vi "iPSset.vi"(7 "Field Rate, T/min":dbl, 8 "error in (no error)":errorcluster, 9 "Target Field, T":dbl, 10 "iPSSetCtrl":T1, 11 "VISA resource name":refnum<visa-resource-name>) -> (0 "error out":errorcluster, 1 "read buffer":string, 2 "number":dbl, 3 "VISA resource name out":refnum<visa-resource-name>)   [LabVIEW 2021]
uses:
  controls/iPSsetCtrl.ctl
  <vilib>/regexp/Match Regular Expression.xnode
panel:
  out "call chain":string[](array[string])
  out "concatenated string 2":string
  out "concatenated string":string
  out "after match":string
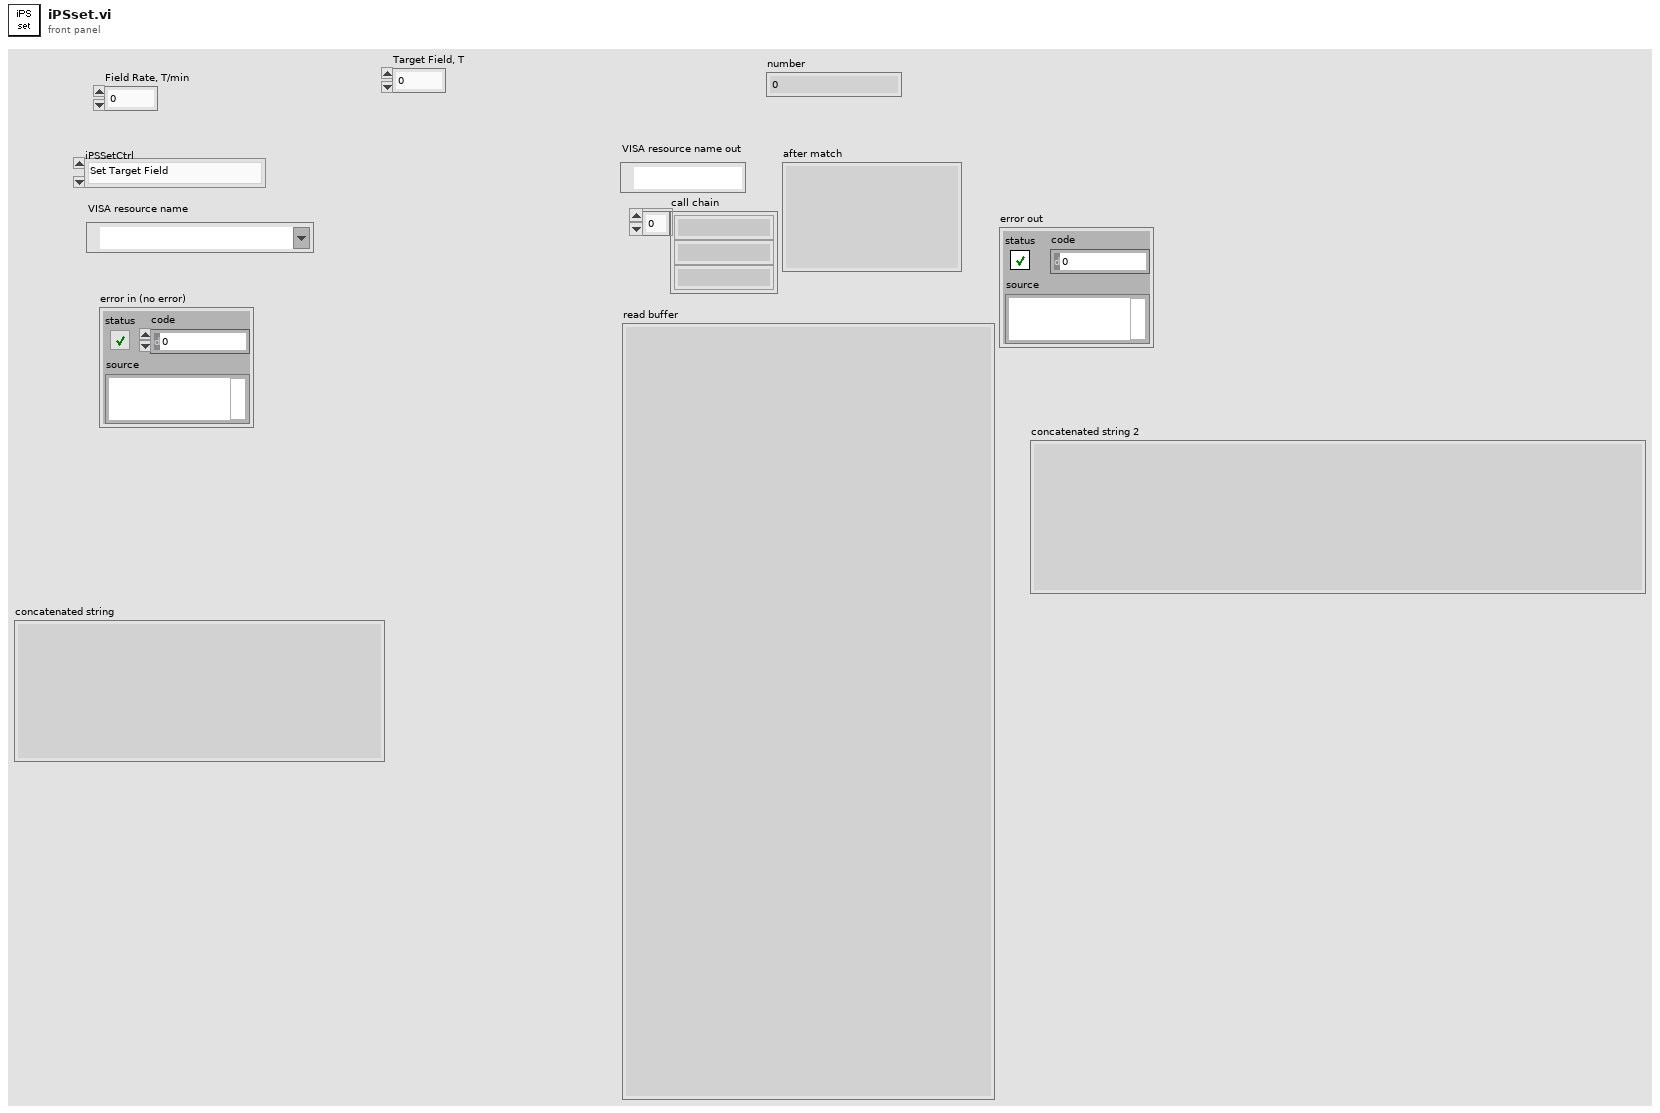
[diagram p1: front panel]
types:
  T1 = typedef "iPSsetCtrl.ctl" = enum16{"Set Target Field", "Set Target Field Rate", "Switch Heater ON", "Switch Heater OFF", "Go to Field", "Go to Zero", "Hold"}
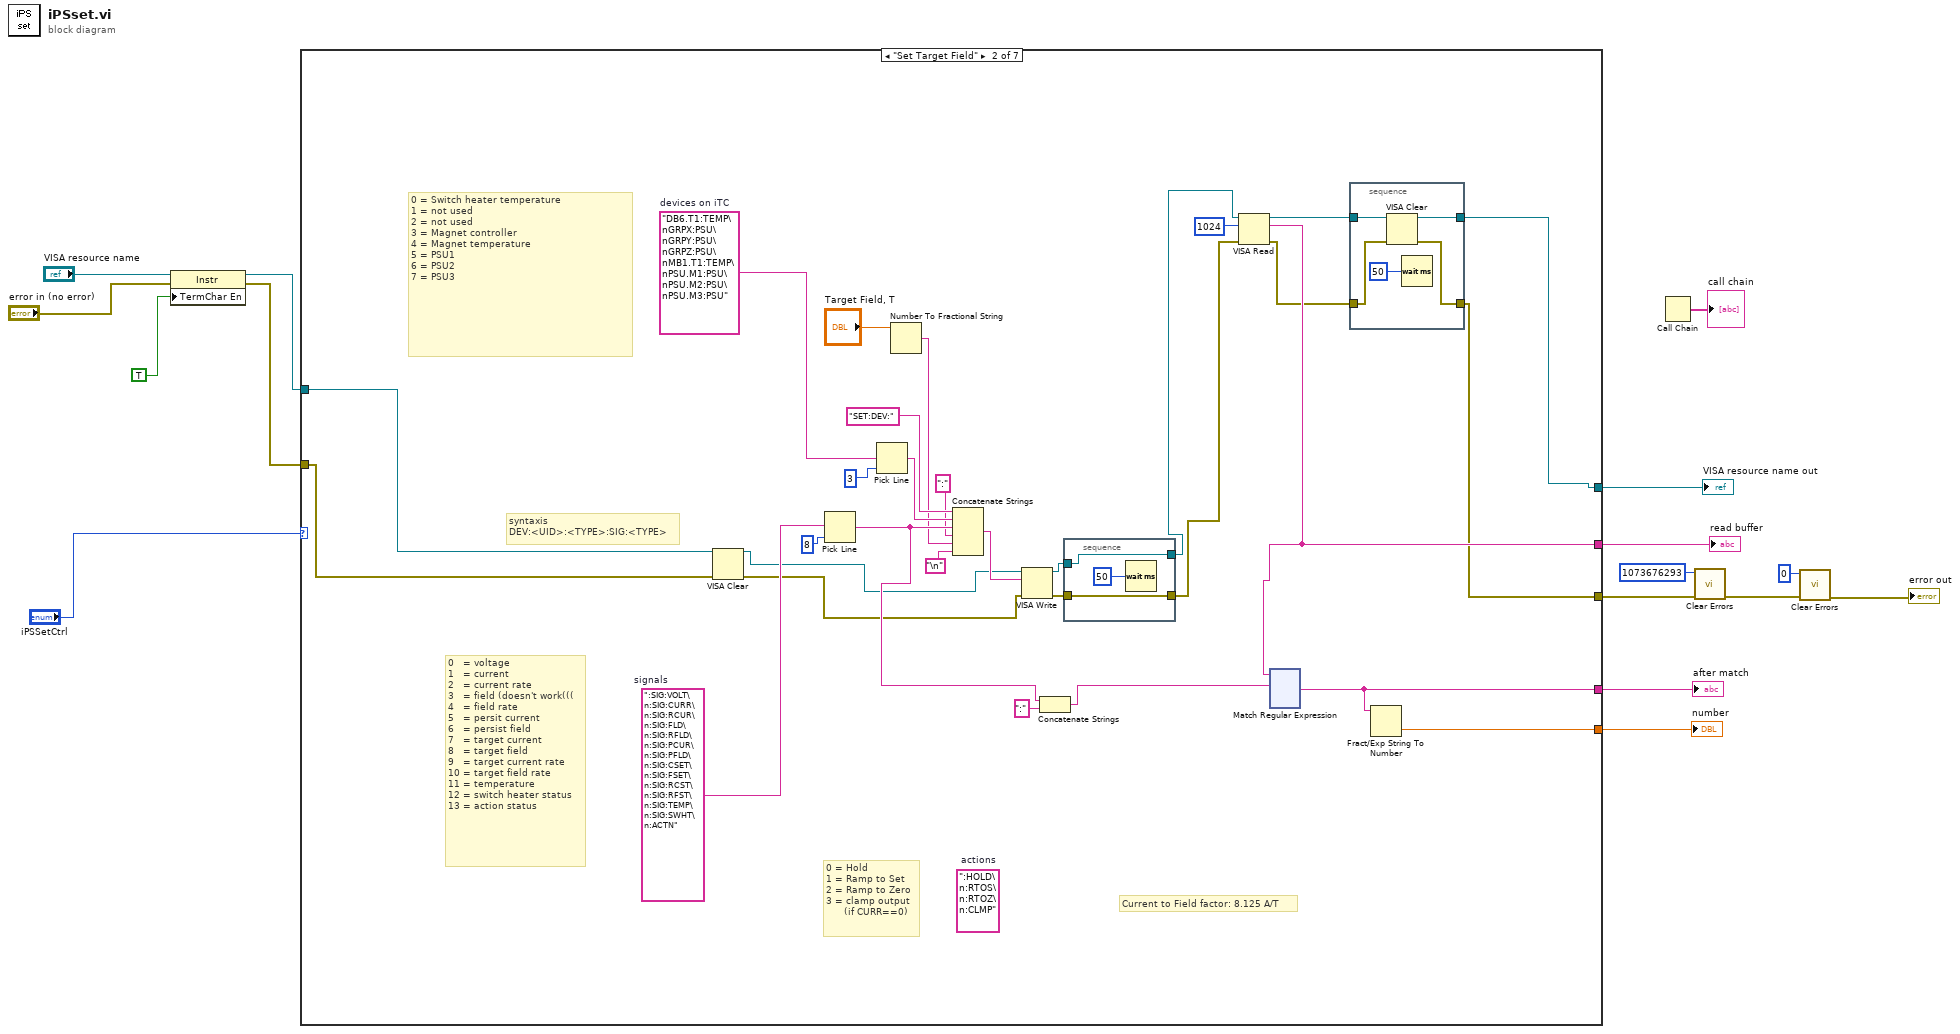
[diagram p0: block diagram]
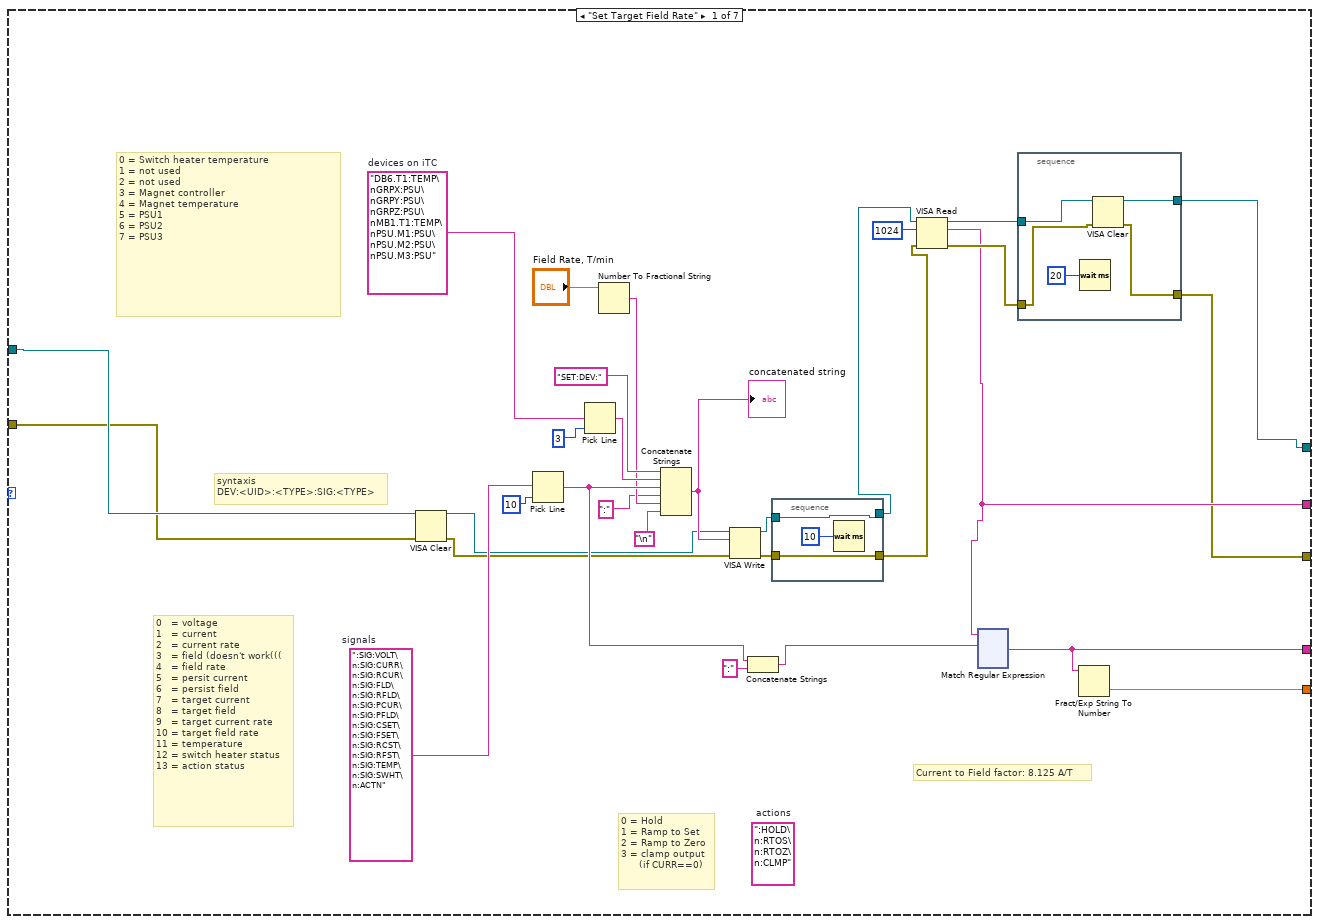
[diagram p2: hidden frame]
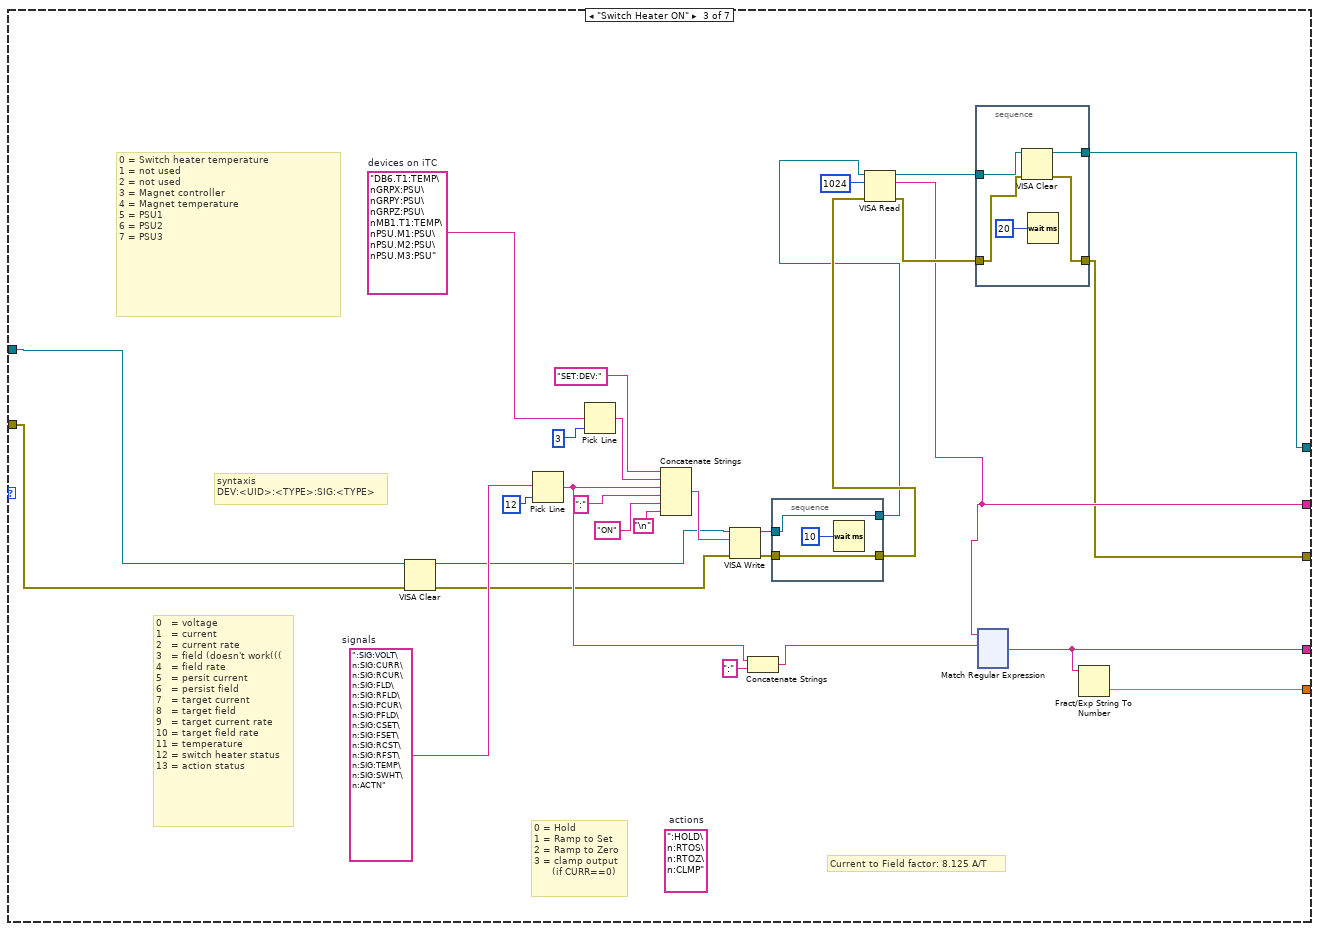
[diagram p3: hidden frame]
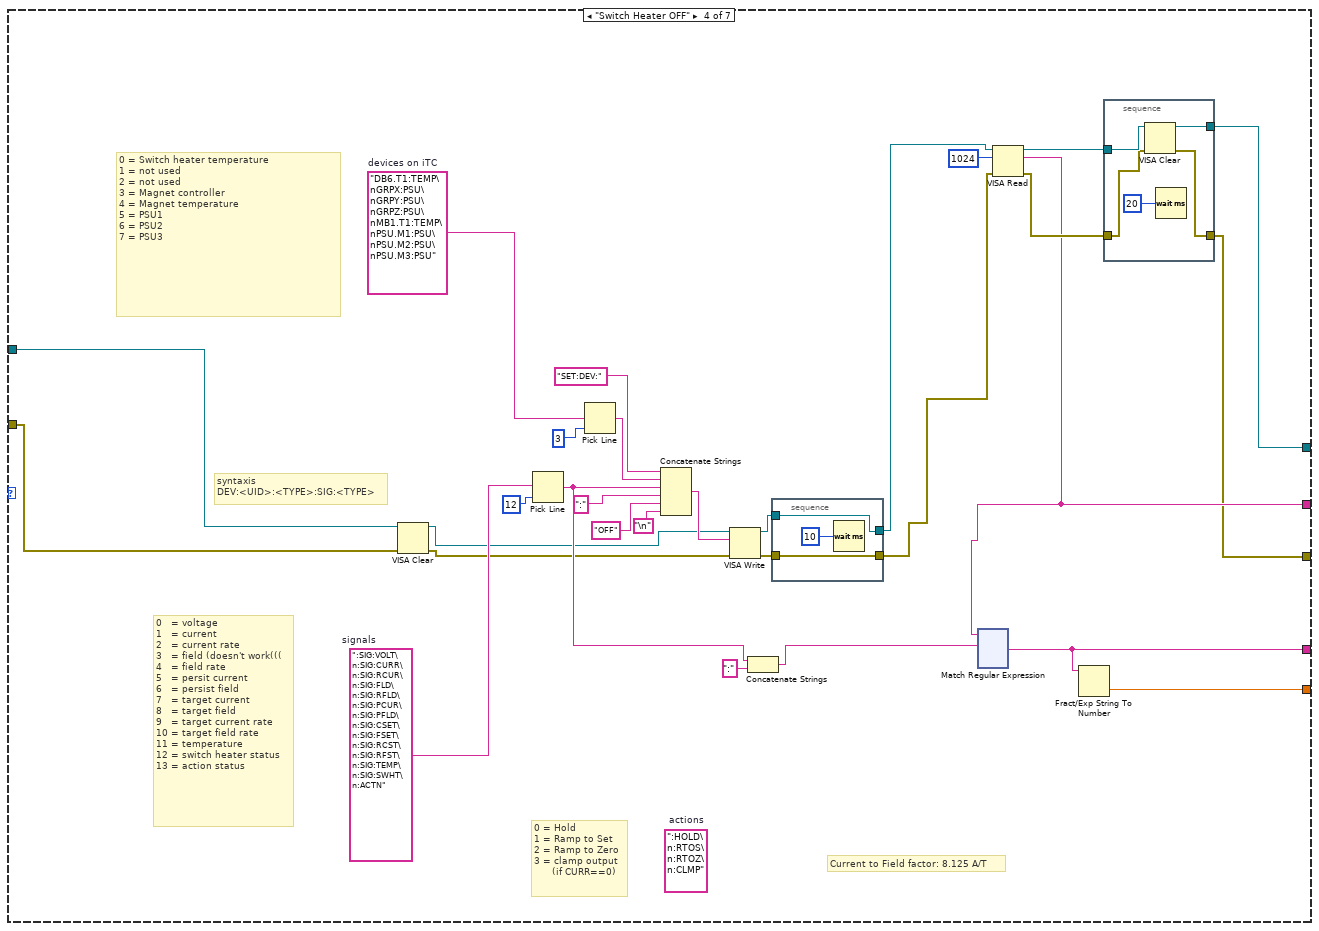
[diagram p4: hidden frame]
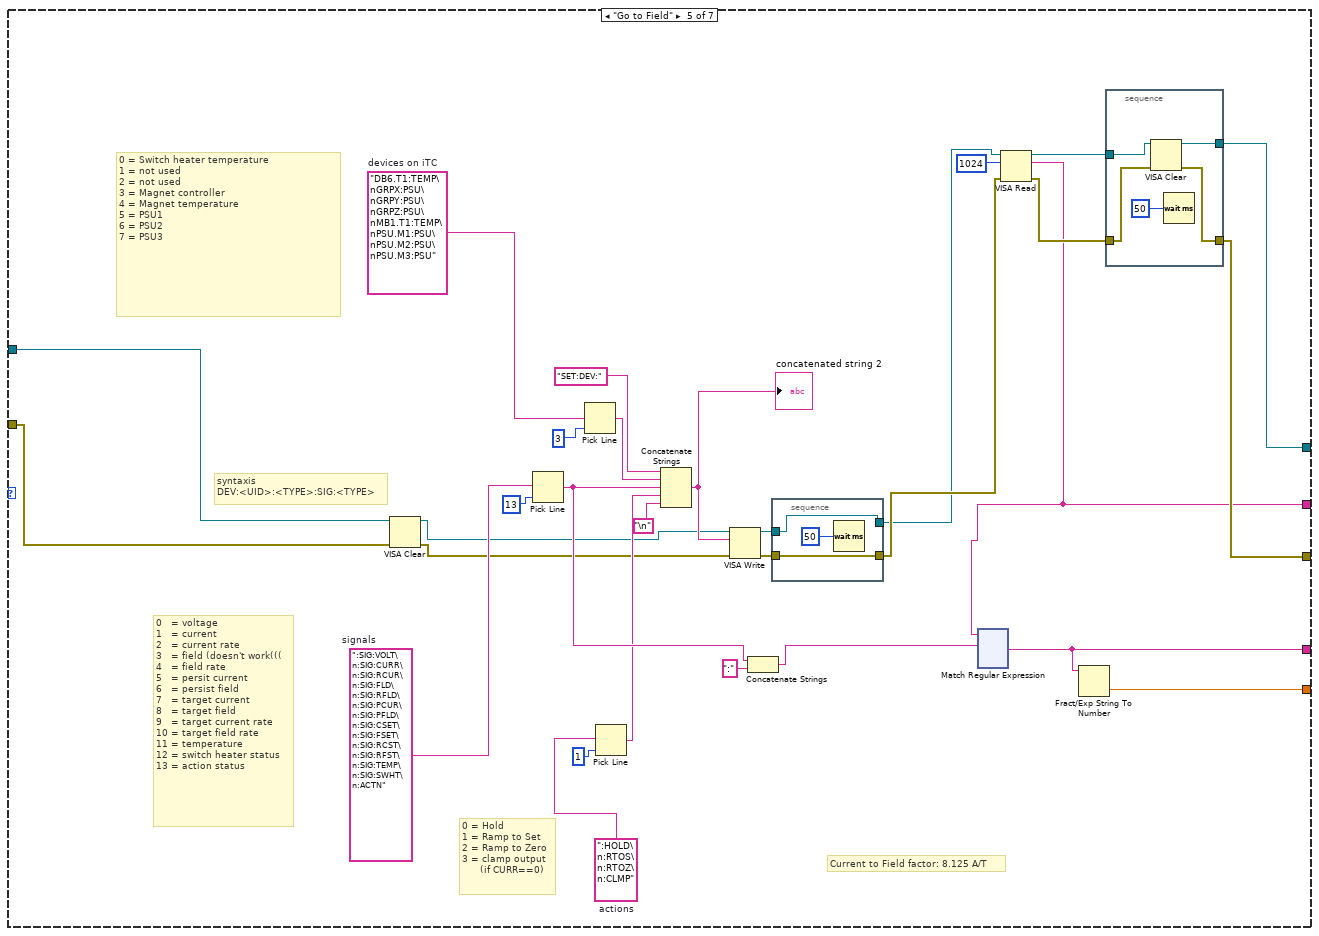
[diagram p5: hidden frame]
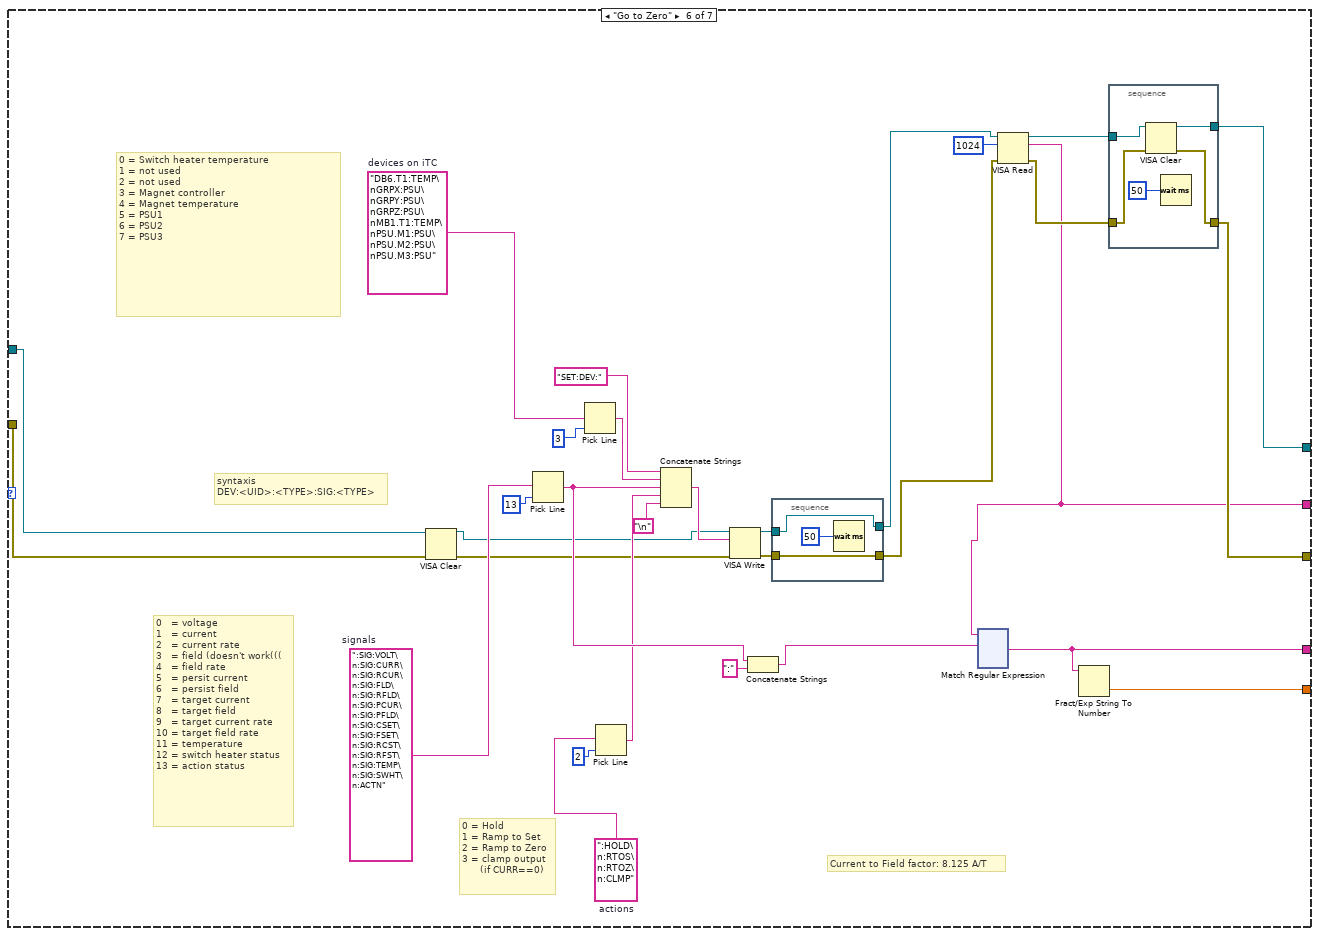
[diagram p6: hidden frame]
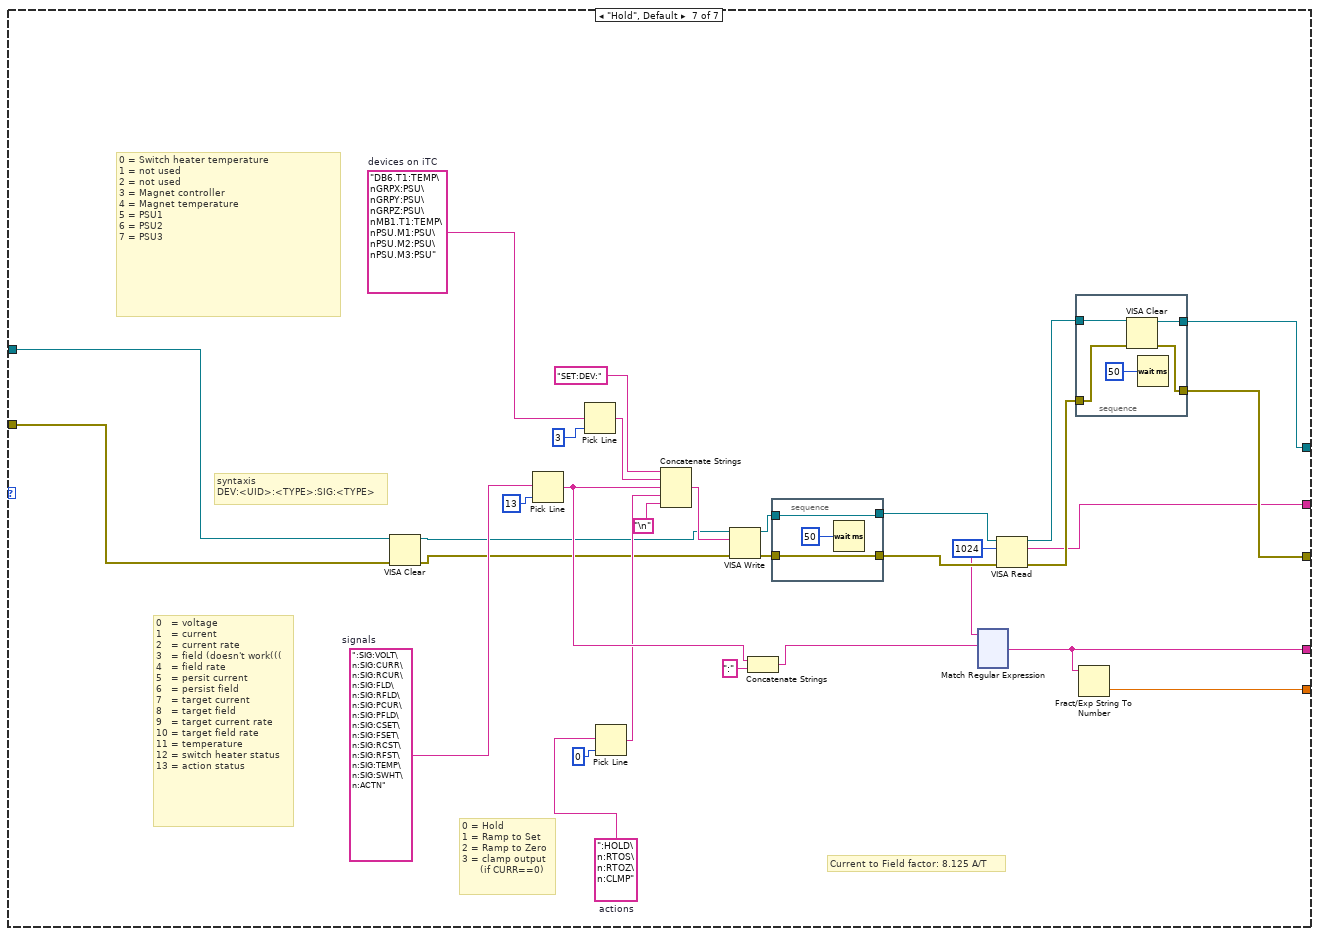
[diagram p7: hidden frame]
diagram:
  n1 = property class="Instr"(reference="VISA resource name", error in="error in (no error)", "TermChar En"=TRUE ("Message Based Settings:Termination Character Enable")) -> (reference out=w10:refnum<visa-resource-name>, error out=w9:errorcluster)
  n2 = case shown="\"Set Target Field\"" "iPSSetCtrl" {
    tunnel: [w25 w180 w335 w489 w645 w800 w954] -> w6
    tunnel: [w19 w174 w329 w483 w637 w793 w947] -> w16
    tunnel: [w26 w182 w336 w490 w644 w798 w953] -> w15
    tunnel: [w36 w191 w345 w499 w654 w809 w964] -> w14
    tunnel: [w35 w190 w344 w498 w653 w808 w963] -> w13
    tunnel: w9 -> [w23 w178 w333 w488 w642 w797 w952]
    tunnel: w10 -> [w24 w179 w334 w485 w640 w794 w949]
    frame "Set Target Field Rate" {
      (unwired) ":HOLD\n:RTOS\n:RTOZ\n:CLMP"  # actions
      w41 = ":SIG:VOLT\n:SIG:CURR\n:SIG:RCUR\n:SIG:FLD\n:SIG:RFLD\n:SIG:PCUR\n:SIG:PFLD\n:SIG:CSET\n:SIG:FSET\n:SIG:RCST\n:SIG:RFST\n:SIG:TEMP\n:SIG:SWHT\n:ACTN"  # signals
      w46 = "DB6.T1:TEMP\nGRPX:PSU\nGRPY:PSU\nGRPZ:PSU\nMB1.T1:TEMP\nPSU.M1:PSU\nPSU.M2:PSU\nPSU.M3:PSU"  # devices on iTC
      # "0 = Hold\n1 = Ramp to Set\n2 = Ramp to Zero\n3 = clamp output\n      (if CURR==0)"
      # "Current to Field factor: 8.125 A/T"
      # "0 = Switch heater temperature\n1 = not used\n2 = not used\n3 = Magnet controller \n4 = Magnet temperature\n5 = PSU1 \n6 = PSU2\n7 = PSU3"
      # "0   = voltage\n1   = current\n2   = current rate\n3   = field (doesn't work(((\n4   = field rate\n5   = persit current\n6   = persist field\n7   = target current\n8   = target field\n9   = target current rate\n10 = target field rate \n11 = temperature\n12 = switch heater status\n13 = action status"
      # "syntaxis\nDEV:<UID>:<TYPE>:SIG:<TYPE>"
      n3 = VISA Clear(VISA resource name=w24, error in (no error)=w23) -> (VISA resource name out=w21:refnum<visa-resource-name>, error out=w22:errorcluster)
      n4 = Pick Line(multi-line string=w41, line index=10) -> (output string=w39:string)  [unwired: 1 in]
      n5 = Pick Line(multi-line string=w46, line index=3) -> (output string=w43:string)  [unwired: 1 in]
      n6 = Number To Fractional String(number="Field Rate, T/min") -> (F-format string=w31:string)  [unwired: 3 in]
      n7 = Concatenate Strings("SET:DEV:" ("write buffer"), w43, w39, ":" ("string"), w31, "\n") -> (w37:string)
      "concatenated string" <- w37
      n8 = VISA Write(VISA resource name=w21, write buffer=w37, error in (no error)=w22) -> (VISA resource name out=w18:refnum<visa-resource-name>, error out=w45:errorcluster)  [unwired: 1 out]
      n9 = Concatenate Strings(w39, ":" ("string")) -> (w38:string)
      n10 = stacked-sequence {
        tunnel: w45 -> [w171]
        tunnel: [w171] -> w27
        tunnel: w18 -> [w169]
        tunnel: [w169] -> w17
        frame #0 {
          n11 = Wait (ms)(milliseconds to wait=u32 10) -> ()  [unwired: 1 out]
        }
      }
      n12 = VISA Read(VISA resource name=w17, byte count=u32 1024, error in (no error)=w27) -> (VISA resource name out=w20:refnum<visa-resource-name>, read buffer=w26:string, error out=w29:errorcluster)  [unwired: 1 out]
      n13 = xnode "Match Regular Expression"("input string"=w26, "regular expression"=w38) -> ("after match"=w36:string)  [unwired: 4 in, 4 out]
      n14 = stacked-sequence {
        tunnel: [w48] -> w25
        tunnel: w29 -> [w47]
        tunnel: w20 -> [w50]
        tunnel: [w49] -> w19
        frame #0 {
          n15 = Wait (ms)(milliseconds to wait=u32 20) -> ()  [unwired: 1 out]
          n16 = VISA Clear(VISA resource name=w50, error in (no error)=w47) -> (VISA resource name out=w49:refnum<visa-resource-name>, error out=w48:errorcluster)
        }
      }
      n17 = Fract/Exp String To Number(string=w36) -> (number=w35:dbl)  [unwired: 3 in, 1 out]
    }
    frame "Set Target Field" {
      (unwired) ":HOLD\n:RTOS\n:RTOZ\n:CLMP"  # actions
      w196 = ":SIG:VOLT\n:SIG:CURR\n:SIG:RCUR\n:SIG:FLD\n:SIG:RFLD\n:SIG:PCUR\n:SIG:PFLD\n:SIG:CSET\n:SIG:FSET\n:SIG:RCST\n:SIG:RFST\n:SIG:TEMP\n:SIG:SWHT\n:ACTN"  # signals
      w201 = "DB6.T1:TEMP\nGRPX:PSU\nGRPY:PSU\nGRPZ:PSU\nMB1.T1:TEMP\nPSU.M1:PSU\nPSU.M2:PSU\nPSU.M3:PSU"  # devices on iTC
      # "0 = Hold\n1 = Ramp to Set\n2 = Ramp to Zero\n3 = clamp output\n      (if CURR==0)"
      # "Current to Field factor: 8.125 A/T"
      # "0 = Switch heater temperature\n1 = not used\n2 = not used\n3 = Magnet controller \n4 = Magnet temperature\n5 = PSU1 \n6 = PSU2\n7 = PSU3"
      # "0   = voltage\n1   = current\n2   = current rate\n3   = field (doesn't work(((\n4   = field rate\n5   = persit current\n6   = persist field\n7   = target current\n8   = target field\n9   = target current rate\n10 = target field rate \n11 = temperature\n12 = switch heater status\n13 = action status"
      # "syntaxis\nDEV:<UID>:<TYPE>:SIG:<TYPE>"
      n18 = VISA Clear(VISA resource name=w179, error in (no error)=w178) -> (VISA resource name out=w176:refnum<visa-resource-name>, error out=w177:errorcluster)
      n19 = Pick Line(multi-line string=w196, line index=8) -> (output string=w194:string)  [unwired: 1 in]
      n20 = Pick Line(multi-line string=w201, line index=3) -> (output string=w198:string)  [unwired: 1 in]
      n21 = Number To Fractional String(number="Target Field, T") -> (F-format string=w186:string)  [unwired: 3 in]
      n22 = Concatenate Strings("SET:DEV:" ("write buffer"), w198, w194, ":" ("string"), w186, "\n") -> (w192:string)
      n23 = VISA Write(VISA resource name=w176, write buffer=w192, error in (no error)=w177) -> (VISA resource name out=w173:refnum<visa-resource-name>, error out=w200:errorcluster)  [unwired: 1 out]
      n24 = Concatenate Strings(w194, ":" ("string")) -> (w193:string)
      n25 = stacked-sequence {
        tunnel: w200 -> [w326]
        tunnel: [w326] -> w183
        tunnel: w173 -> [w324]
        tunnel: [w324] -> w172
        frame #0 {
          n26 = Wait (ms)(milliseconds to wait=u32 50) -> ()  [unwired: 1 out]
        }
      }
      n27 = VISA Read(VISA resource name=w172, byte count=u32 1024, error in (no error)=w183) -> (VISA resource name out=w175:refnum<visa-resource-name>, read buffer=w182:string, error out=w181:errorcluster)  [unwired: 1 out]
      n28 = xnode "Match Regular Expression"("input string"=w182, "regular expression"=w193) -> ("after match"=w191:string)  [unwired: 4 in, 4 out]
      n29 = stacked-sequence {
        tunnel: w181 -> [w204]
        tunnel: [w203] -> w180
        tunnel: w175 -> [w205]
        tunnel: [w202] -> w174
        frame #0 {
          n30 = VISA Clear(VISA resource name=w205, error in (no error)=w204) -> (VISA resource name out=w202:refnum<visa-resource-name>, error out=w203:errorcluster)
          n31 = Wait (ms)(milliseconds to wait=u32 50) -> ()  [unwired: 1 out]
        }
      }
      n32 = Fract/Exp String To Number(string=w191) -> (number=w190:dbl)  [unwired: 3 in, 1 out]
    }
    frame "Switch Heater ON" {
      (unwired) ":HOLD\n:RTOS\n:RTOZ\n:CLMP"  # actions
      w350 = ":SIG:VOLT\n:SIG:CURR\n:SIG:RCUR\n:SIG:FLD\n:SIG:RFLD\n:SIG:PCUR\n:SIG:PFLD\n:SIG:CSET\n:SIG:FSET\n:SIG:RCST\n:SIG:RFST\n:SIG:TEMP\n:SIG:SWHT\n:ACTN"  # signals
      w355 = "DB6.T1:TEMP\nGRPX:PSU\nGRPY:PSU\nGRPZ:PSU\nMB1.T1:TEMP\nPSU.M1:PSU\nPSU.M2:PSU\nPSU.M3:PSU"  # devices on iTC
      # "0 = Hold\n1 = Ramp to Set\n2 = Ramp to Zero\n3 = clamp output\n      (if CURR==0)"
      # "Current to Field factor: 8.125 A/T"
      # "0 = Switch heater temperature\n1 = not used\n2 = not used\n3 = Magnet controller \n4 = Magnet temperature\n5 = PSU1 \n6 = PSU2\n7 = PSU3"
      # "0   = voltage\n1   = current\n2   = current rate\n3   = field (doesn't work(((\n4   = field rate\n5   = persit current\n6   = persist field\n7   = target current\n8   = target field\n9   = target current rate\n10 = target field rate \n11 = temperature\n12 = switch heater status\n13 = action status"
      # "syntaxis\nDEV:<UID>:<TYPE>:SIG:<TYPE>"
      n33 = VISA Clear(VISA resource name=w334, error in (no error)=w333) -> (VISA resource name out=w331:refnum<visa-resource-name>, error out=w332:errorcluster)
      n34 = Pick Line(multi-line string=w350, line index=12) -> (output string=w348:string)  [unwired: 1 in]
      n35 = Pick Line(multi-line string=w355, line index=3) -> (output string=w352:string)  [unwired: 1 in]
      n36 = Concatenate Strings("SET:DEV:" ("write buffer"), w352, w348, ":" ("string"), "ON" ("string"), "\n") -> (w346:string)
      n37 = VISA Write(VISA resource name=w331, write buffer=w346, error in (no error)=w332) -> (VISA resource name out=w327:refnum<visa-resource-name>, error out=w354:errorcluster)  [unwired: 1 out]
      n38 = Concatenate Strings(w348, ":" ("string")) -> (w347:string)
      n39 = stacked-sequence {
        tunnel: w354 -> [w480]
        tunnel: [w480] -> w337
        tunnel: [w478] -> w328
        tunnel: w327 -> [w478]
        frame #0 {
          n40 = Wait (ms)(milliseconds to wait=u32 10) -> ()  [unwired: 1 out]
        }
      }
      n41 = VISA Read(VISA resource name=w328, byte count=u32 1024, error in (no error)=w337) -> (VISA resource name out=w330:refnum<visa-resource-name>, read buffer=w336:string, error out=w338:errorcluster)  [unwired: 1 out]
      n42 = stacked-sequence {
        tunnel: w338 -> [w356]
        tunnel: [w357] -> w335
        tunnel: w330 -> [w359]
        tunnel: [w358] -> w329
        frame #0 {
          n43 = VISA Clear(VISA resource name=w359, error in (no error)=w356) -> (VISA resource name out=w358:refnum<visa-resource-name>, error out=w357:errorcluster)
          n44 = Wait (ms)(milliseconds to wait=u32 20) -> ()  [unwired: 1 out]
        }
      }
      n45 = xnode "Match Regular Expression"("input string"=w336, "regular expression"=w347) -> ("after match"=w345:string)  [unwired: 4 in, 4 out]
      n46 = Fract/Exp String To Number(string=w345) -> (number=w344:dbl)  [unwired: 3 in, 1 out]
    }
    frame "Switch Heater OFF" {
      (unwired) ":HOLD\n:RTOS\n:RTOZ\n:CLMP"  # actions
      w504 = ":SIG:VOLT\n:SIG:CURR\n:SIG:RCUR\n:SIG:FLD\n:SIG:RFLD\n:SIG:PCUR\n:SIG:PFLD\n:SIG:CSET\n:SIG:FSET\n:SIG:RCST\n:SIG:RFST\n:SIG:TEMP\n:SIG:SWHT\n:ACTN"  # signals
      w509 = "DB6.T1:TEMP\nGRPX:PSU\nGRPY:PSU\nGRPZ:PSU\nMB1.T1:TEMP\nPSU.M1:PSU\nPSU.M2:PSU\nPSU.M3:PSU"  # devices on iTC
      # "0 = Hold\n1 = Ramp to Set\n2 = Ramp to Zero\n3 = clamp output\n      (if CURR==0)"
      # "Current to Field factor: 8.125 A/T"
      # "0 = Switch heater temperature\n1 = not used\n2 = not used\n3 = Magnet controller \n4 = Magnet temperature\n5 = PSU1 \n6 = PSU2\n7 = PSU3"
      # "0   = voltage\n1   = current\n2   = current rate\n3   = field (doesn't work(((\n4   = field rate\n5   = persit current\n6   = persist field\n7   = target current\n8   = target field\n9   = target current rate\n10 = target field rate \n11 = temperature\n12 = switch heater status\n13 = action status"
      # "syntaxis\nDEV:<UID>:<TYPE>:SIG:<TYPE>"
      n47 = VISA Clear(VISA resource name=w485, error in (no error)=w488) -> (VISA resource name out=w486:refnum<visa-resource-name>, error out=w487:errorcluster)
      n48 = Pick Line(multi-line string=w504, line index=12) -> (output string=w502:string)  [unwired: 1 in]
      n49 = Pick Line(multi-line string=w509, line index=3) -> (output string=w506:string)  [unwired: 1 in]
      n50 = Concatenate Strings("SET:DEV:" ("write buffer"), w506, w502, ":" ("string"), "OFF" ("string"), "\n") -> (w500:string)
      n51 = VISA Write(VISA resource name=w486, write buffer=w500, error in (no error)=w487) -> (VISA resource name out=w482:refnum<visa-resource-name>, error out=w508:errorcluster)  [unwired: 1 out]
      n52 = Concatenate Strings(w502, ":" ("string")) -> (w501:string)
      n53 = stacked-sequence {
        tunnel: w508 -> [w634]
        tunnel: [w634] -> w491
        tunnel: [w632] -> w481
        tunnel: w482 -> [w632]
        frame #0 {
          n54 = Wait (ms)(milliseconds to wait=u32 10) -> ()  [unwired: 1 out]
        }
      }
      n55 = VISA Read(VISA resource name=w481, byte count=u32 1024, error in (no error)=w491) -> (VISA resource name out=w484:refnum<visa-resource-name>, read buffer=w490:string, error out=w492:errorcluster)  [unwired: 1 out]
      n56 = xnode "Match Regular Expression"("input string"=w490, "regular expression"=w501) -> ("after match"=w499:string)  [unwired: 4 in, 4 out]
      n57 = Fract/Exp String To Number(string=w499) -> (number=w498:dbl)  [unwired: 3 in, 1 out]
      n58 = stacked-sequence {
        tunnel: w492 -> [w510]
        tunnel: [w511] -> w489
        tunnel: w484 -> [w513]
        tunnel: [w512] -> w483
        frame #0 {
          n59 = VISA Clear(VISA resource name=w513, error in (no error)=w510) -> (VISA resource name out=w512:refnum<visa-resource-name>, error out=w511:errorcluster)
          n60 = Wait (ms)(milliseconds to wait=u32 20) -> ()  [unwired: 1 out]
        }
      }
    }
    frame "Go to Field" {
      w649 = ":HOLD\n:RTOS\n:RTOZ\n:CLMP"  # actions
      w659 = ":SIG:VOLT\n:SIG:CURR\n:SIG:RCUR\n:SIG:FLD\n:SIG:RFLD\n:SIG:PCUR\n:SIG:PFLD\n:SIG:CSET\n:SIG:FSET\n:SIG:RCST\n:SIG:RFST\n:SIG:TEMP\n:SIG:SWHT\n:ACTN"  # signals
      w664 = "DB6.T1:TEMP\nGRPX:PSU\nGRPY:PSU\nGRPZ:PSU\nMB1.T1:TEMP\nPSU.M1:PSU\nPSU.M2:PSU\nPSU.M3:PSU"  # devices on iTC
      # "0 = Hold\n1 = Ramp to Set\n2 = Ramp to Zero\n3 = clamp output\n      (if CURR==0)"
      # "Current to Field factor: 8.125 A/T"
      # "0 = Switch heater temperature\n1 = not used\n2 = not used\n3 = Magnet controller \n4 = Magnet temperature\n5 = PSU1 \n6 = PSU2\n7 = PSU3"
      # "0   = voltage\n1   = current\n2   = current rate\n3   = field (doesn't work(((\n4   = field rate\n5   = persit current\n6   = persist field\n7   = target current\n8   = target field\n9   = target current rate\n10 = target field rate \n11 = temperature\n12 = switch heater status\n13 = action status"
      # "syntaxis\nDEV:<UID>:<TYPE>:SIG:<TYPE>"
      n61 = VISA Clear(VISA resource name=w640, error in (no error)=w642) -> (VISA resource name out=w639:refnum<visa-resource-name>, error out=w641:errorcluster)
      n62 = Pick Line(multi-line string=w659, line index=13) -> (output string=w657:string)  [unwired: 1 in]
      n63 = Pick Line(multi-line string=w664, line index=3) -> (output string=w661:string)  [unwired: 1 in]
      n64 = Pick Line(multi-line string=w649, line index=1) -> (output string=w648:string)  [unwired: 1 in]
      n65 = Concatenate Strings("SET:DEV:" ("write buffer"), w661, w657, w648, "\n") -> (w655:string)
      "concatenated string 2" <- w655
      n66 = VISA Write(VISA resource name=w639, write buffer=w655, error in (no error)=w641) -> (VISA resource name out=w636:refnum<visa-resource-name>, error out=w663:errorcluster)  [unwired: 1 out]
      n67 = Concatenate Strings(w657, ":" ("string")) -> (w656:string)
      n68 = stacked-sequence {
        tunnel: w663 -> [w789]
        tunnel: [w789] -> w643
        tunnel: w636 -> [w787]
        tunnel: [w787] -> w635
        frame #0 {
          n69 = Wait (ms)(milliseconds to wait=u32 50) -> ()  [unwired: 1 out]
        }
      }
      n70 = VISA Read(VISA resource name=w635, byte count=u32 1024, error in (no error)=w643) -> (VISA resource name out=w638:refnum<visa-resource-name>, read buffer=w644:string, error out=w646:errorcluster)  [unwired: 1 out]
      n71 = xnode "Match Regular Expression"("input string"=w644, "regular expression"=w656) -> ("after match"=w654:string)  [unwired: 4 in, 4 out]
      n72 = Fract/Exp String To Number(string=w654) -> (number=w653:dbl)  [unwired: 3 in, 1 out]
      n73 = stacked-sequence {
        tunnel: w646 -> [w665]
        tunnel: [w666] -> w645
        tunnel: w638 -> [w668]
        tunnel: [w667] -> w637
        frame #0 {
          n74 = VISA Clear(VISA resource name=w668, error in (no error)=w665) -> (VISA resource name out=w667:refnum<visa-resource-name>, error out=w666:errorcluster)
          n75 = Wait (ms)(milliseconds to wait=u32 50) -> ()  [unwired: 1 out]
        }
      }
    }
    frame "Go to Zero" {
      w804 = ":HOLD\n:RTOS\n:RTOZ\n:CLMP"  # actions
      w814 = ":SIG:VOLT\n:SIG:CURR\n:SIG:RCUR\n:SIG:FLD\n:SIG:RFLD\n:SIG:PCUR\n:SIG:PFLD\n:SIG:CSET\n:SIG:FSET\n:SIG:RCST\n:SIG:RFST\n:SIG:TEMP\n:SIG:SWHT\n:ACTN"  # signals
      w819 = "DB6.T1:TEMP\nGRPX:PSU\nGRPY:PSU\nGRPZ:PSU\nMB1.T1:TEMP\nPSU.M1:PSU\nPSU.M2:PSU\nPSU.M3:PSU"  # devices on iTC
      # "0 = Hold\n1 = Ramp to Set\n2 = Ramp to Zero\n3 = clamp output\n      (if CURR==0)"
      # "Current to Field factor: 8.125 A/T"
      # "0 = Switch heater temperature\n1 = not used\n2 = not used\n3 = Magnet controller \n4 = Magnet temperature\n5 = PSU1 \n6 = PSU2\n7 = PSU3"
      # "0   = voltage\n1   = current\n2   = current rate\n3   = field (doesn't work(((\n4   = field rate\n5   = persit current\n6   = persist field\n7   = target current\n8   = target field\n9   = target current rate\n10 = target field rate \n11 = temperature\n12 = switch heater status\n13 = action status"
      # "syntaxis\nDEV:<UID>:<TYPE>:SIG:<TYPE>"
      n76 = VISA Clear(VISA resource name=w794, error in (no error)=w797) -> (VISA resource name out=w795:refnum<visa-resource-name>, error out=w796:errorcluster)
      n77 = Pick Line(multi-line string=w814, line index=13) -> (output string=w812:string)  [unwired: 1 in]
      n78 = Pick Line(multi-line string=w819, line index=3) -> (output string=w816:string)  [unwired: 1 in]
      n79 = Pick Line(multi-line string=w804, line index=2) -> (output string=w803:string)  [unwired: 1 in]
      n80 = Concatenate Strings("SET:DEV:" ("write buffer"), w816, w812, w803, "\n") -> (w810:string)
      n81 = VISA Write(VISA resource name=w795, write buffer=w810, error in (no error)=w796) -> (VISA resource name out=w791:refnum<visa-resource-name>, error out=w818:errorcluster)  [unwired: 1 out]
      n82 = Concatenate Strings(w812, ":" ("string")) -> (w811:string)
      n83 = stacked-sequence {
        tunnel: w818 -> [w944]
        tunnel: [w944] -> w799
        tunnel: w791 -> [w942]
        tunnel: [w942] -> w790
        frame #0 {
          n84 = Wait (ms)(milliseconds to wait=u32 50) -> ()  [unwired: 1 out]
        }
      }
      n85 = VISA Read(VISA resource name=w790, byte count=u32 1024, error in (no error)=w799) -> (VISA resource name out=w792:refnum<visa-resource-name>, read buffer=w798:string, error out=w801:errorcluster)  [unwired: 1 out]
      n86 = xnode "Match Regular Expression"("input string"=w798, "regular expression"=w811) -> ("after match"=w809:string)  [unwired: 4 in, 4 out]
      n87 = Fract/Exp String To Number(string=w809) -> (number=w808:dbl)  [unwired: 3 in, 1 out]
      n88 = stacked-sequence {
        tunnel: w801 -> [w821]
        tunnel: [w820] -> w800
        tunnel: [w823] -> w793
        tunnel: w792 -> [w822]
        frame #0 {
          n89 = VISA Clear(VISA resource name=w822, error in (no error)=w821) -> (VISA resource name out=w823:refnum<visa-resource-name>, error out=w820:errorcluster)
          n90 = Wait (ms)(milliseconds to wait=u32 50) -> ()  [unwired: 1 out]
        }
      }
    }
    frame "Hold", Default {
      w959 = ":HOLD\n:RTOS\n:RTOZ\n:CLMP"  # actions
      w969 = ":SIG:VOLT\n:SIG:CURR\n:SIG:RCUR\n:SIG:FLD\n:SIG:RFLD\n:SIG:PCUR\n:SIG:PFLD\n:SIG:CSET\n:SIG:FSET\n:SIG:RCST\n:SIG:RFST\n:SIG:TEMP\n:SIG:SWHT\n:ACTN"  # signals
      w974 = "DB6.T1:TEMP\nGRPX:PSU\nGRPY:PSU\nGRPZ:PSU\nMB1.T1:TEMP\nPSU.M1:PSU\nPSU.M2:PSU\nPSU.M3:PSU"  # devices on iTC
      # "0 = Hold\n1 = Ramp to Set\n2 = Ramp to Zero\n3 = clamp output\n      (if CURR==0)"
      # "Current to Field factor: 8.125 A/T"
      # "0 = Switch heater temperature\n1 = not used\n2 = not used\n3 = Magnet controller \n4 = Magnet temperature\n5 = PSU1 \n6 = PSU2\n7 = PSU3"
      # "0   = voltage\n1   = current\n2   = current rate\n3   = field (doesn't work(((\n4   = field rate\n5   = persit current\n6   = persist field\n7   = target current\n8   = target field\n9   = target current rate\n10 = target field rate \n11 = temperature\n12 = switch heater status\n13 = action status"
      # "syntaxis\nDEV:<UID>:<TYPE>:SIG:<TYPE>"
      n91 = VISA Clear(VISA resource name=w949, error in (no error)=w952) -> (VISA resource name out=w950:refnum<visa-resource-name>, error out=w951:errorcluster)
      n92 = Pick Line(multi-line string=w969, line index=13) -> (output string=w967:string)  [unwired: 1 in]
      n93 = Pick Line(multi-line string=w974, line index=3) -> (output string=w971:string)  [unwired: 1 in]
      n94 = Pick Line(multi-line string=w959, line index=0) -> (output string=w958:string)  [unwired: 1 in]
      n95 = Concatenate Strings("SET:DEV:" ("write buffer"), w971, w967, w958, "\n") -> (w965:string)
      n96 = VISA Write(VISA resource name=w950, write buffer=w965, error in (no error)=w951) -> (VISA resource name out=w946:refnum<visa-resource-name>, error out=w973:errorcluster)  [unwired: 1 out]
      n97 = Concatenate Strings(w967, ":" ("string")) -> (w966:string)
      n98 = stacked-sequence {
        tunnel: w973 -> [w1099]
        tunnel: [w1099] -> w956
        tunnel: [w1097] -> w945
        tunnel: w946 -> [w1097]
        frame #0 {
          n99 = Wait (ms)(milliseconds to wait=u32 50) -> ()  [unwired: 1 out]
        }
      }
      n100 = VISA Read(VISA resource name=w945, byte count=u32 1024, error in (no error)=w956) -> (VISA resource name out=w948:refnum<visa-resource-name>, read buffer=w953:string, error out=w955:errorcluster)  [unwired: 1 out]
      n101 = xnode "Match Regular Expression"("input string"=w953, "regular expression"=w966) -> ("after match"=w964:string)  [unwired: 4 in, 4 out]
      n102 = stacked-sequence {
        tunnel: [w976] -> w954
        tunnel: w955 -> [w977]
        tunnel: w948 -> [w978]
        tunnel: [w975] -> w947
        frame #0 {
          n103 = VISA Clear(VISA resource name=w978, error in (no error)=w977) -> (VISA resource name out=w975:refnum<visa-resource-name>, error out=w976:errorcluster)
          n104 = Wait (ms)(milliseconds to wait=u32 50) -> ()  [unwired: 1 out]
        }
      }
      n105 = Fract/Exp String To Number(string=w964) -> (number=w963:dbl)  [unwired: 3 in, 1 out]
    }
  }
  "read buffer" <- w15
  "VISA resource name out" <- w16
  "after match" <- w14
  "number" <- w13
  n106 = Call Chain() -> (call chain=→"call chain":string[])
  n107 = call <vilib>:"Clear Errors.vi"("error in (no error)"=w6, "specific error code to clear (0: all)"=1073676293) -> ("error out"=w3:errorcluster)  [unwired: 4 in, 1 out]
  n108 = call <vilib>:"Clear Errors.vi"("error in (no error)"=w3, "specific error code to clear (0: all)"=0) -> ("error out"=→"error out":errorcluster)  [unwired: 4 in, 1 out]
